vi "Read HDI Picked.vi"(8 "error in (no error)":errorcluster, 11 "PickerTool Class in":refnum<class "PickerTool Class.lvclass">) -> (0 "error out":errorcluster, 2 "HDI Picked":bool, 3 "PickerTool Class out":refnum<class "PickerTool Class.lvclass">)   [LabVIEW 2017, in "PickerTool Class.lvclass"]
uses:
  PickerTool Class.lvclass
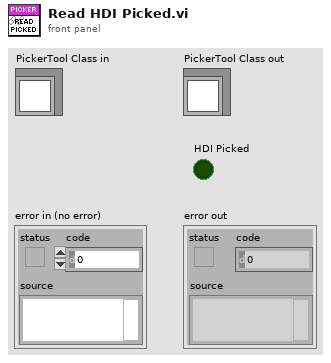
[diagram p1: front panel]
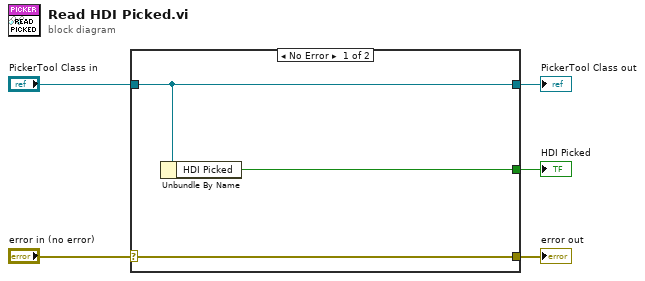
[diagram p0: block diagram]
diagram:
  n1 = case shown="No Error" "error in (no error)" {
    selector: "error in (no error)" -> [w8 w9]
    tunnel: [w8 w9] -> w4
    tunnel: [w7 w10] -> w2
    tunnel: "PickerTool Class in" -> [w7 w10]
    tunnel: [w6 _] -> w1
    frame No Error {
      n2 = Unbundle By Name(w7) -> ("HDI Picked"=w6:bool)
    }
    frame Error {
    }
  }
  "error out" <- w4
  "PickerTool Class out" <- w2
  "HDI Picked" <- w1
